vi "list_subtable_keys.vi"(7 "subtables":string[](array[string]), 8 "error in (no error)":errorcluster, 11 "toml in":refnum<class "toml.lvclass">) -> (0 "error out":errorcluster, 1 "keys":string[](array[string]), 2 "subtable found?":bool, 3 "toml out":refnum<class "toml.lvclass">)   [LabVIEW 2020, in "toml.lvclass"]
uses:
  toml.lvclass
  toml.lvclass/toml.ctl
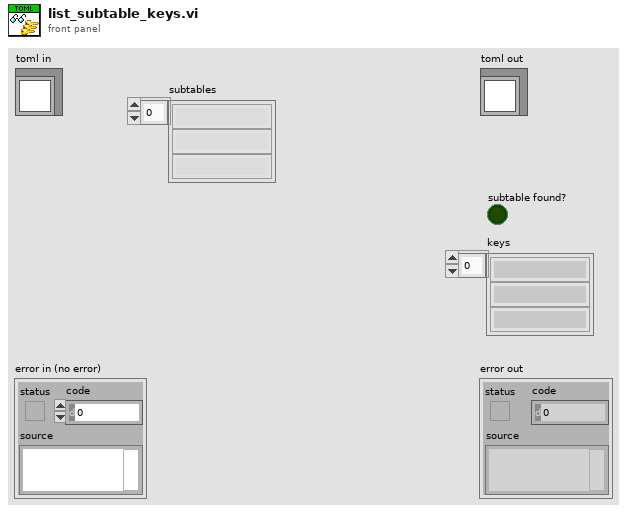
[diagram p1: front panel]
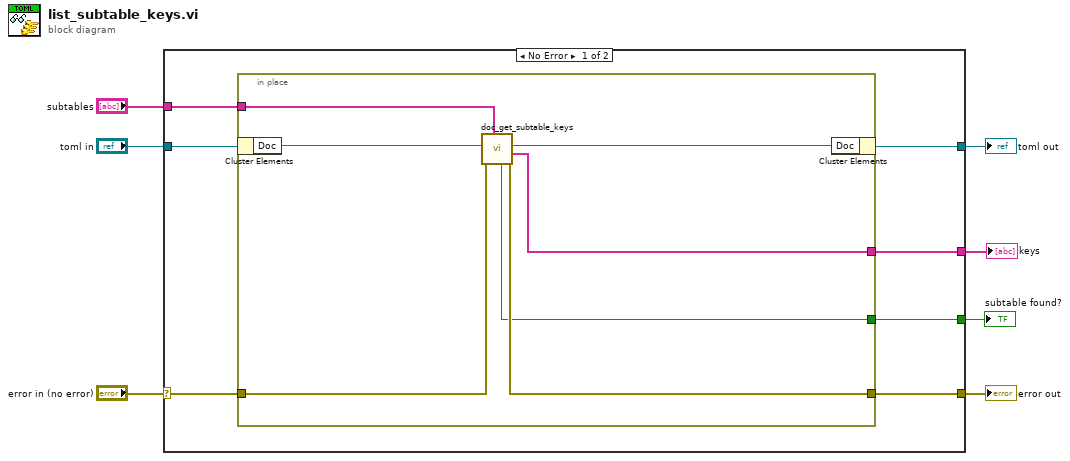
[diagram p0: block diagram]
diagram:
  n1 = case shown="No Error" "error in (no error)" {
    selector: "error in (no error)" -> [w10 w23]
    tunnel: [w11 w23] -> w6
    tunnel: [w13 w22] -> w4
    tunnel: "toml in" -> [w14 w22]
    tunnel: "subtables" -> [w12 _]
    tunnel: [w9 _] -> w2
    tunnel: [w8 _] -> w1
    frame No Error {
      n2 = in-place {
        in-place-border: w12 -> [w19]
        in-place-border: [w20] -> w11
        in-place-border: w10 -> [w21]
        in-place-border: [w15] -> w9
        in-place-border: [w16] -> w8
        n3 = in-place-cluster #1(w14) -> ("Doc"=w18:refnum<class "Doc.lvclass">)
        n4 = call "doc_get_subtable_keys.vi"("subtables"=w19, "error in (no error)"=w21, "Doc in"=w18) -> ("error out"=w20:errorcluster, "keys"=w15:string[], "Doc out"=w17:refnum<class "Doc.lvclass">, "found?"=w16:bool)  [unwired: 5 in]
        n5 = in-place-cluster #1("Doc"=w17) -> (w13:refnum<class "toml.lvclass">)
      }
    }
    frame Error {
    }
  }
  "error out" <- w6
  "toml out" <- w4
  "keys" <- w2
  "subtable found?" <- w1
